vi "Compute if Should Span.vi"(10 "Log Start Time":timestamp, 11 "File Log Specification":T1={"Directory"=path "", "Groups"=[], "Buffer Size"=0, "Properties"=[], "Pretrigger"=FALSE, "Pretrigger Samples"=0, "Name"="", "Timestamp"=FALSE, "Error"=0, "Auto Open"=FALSE, "File Node Ref"=18446744073709551615, "Archive"=FALSE, "Archive Directory"=path "", "Segment Files"=FALSE, "Segment Files By"=enum."Time", "Segment Size"=100000, "Flushed Data Size Total"=0, "Append Waveform Properties"=FALSE, "Logging State"=enum."Not Started", "First Sample Start Time"=timestamp(0 s since 1904-01-01), "System dt"=0.0} {"File Node Ref" format="%.0x"}) -> (3 "Span File":bool)   [LabVIEW 2027, in "Embedded Data Logger Engine.lvlib"]
uses:
  Embedded Data Logger Engine.lvlib
  File Logging Specification.ctl
  Group Logging Specification.ctl
  Group Buffer Data.ctl
  Property Specification.ctl
  <vilib>/NI VeriStand/Custom Device API/Custom Device Item Ref.ctl
  Shared/Segment Files By.ctl
  Logging State.ctl
  <vilib>/NI VeriStand/Custom Device API/Custom Device API.lvlib
  Shared/Embedded Data Logger Shared.lvlib
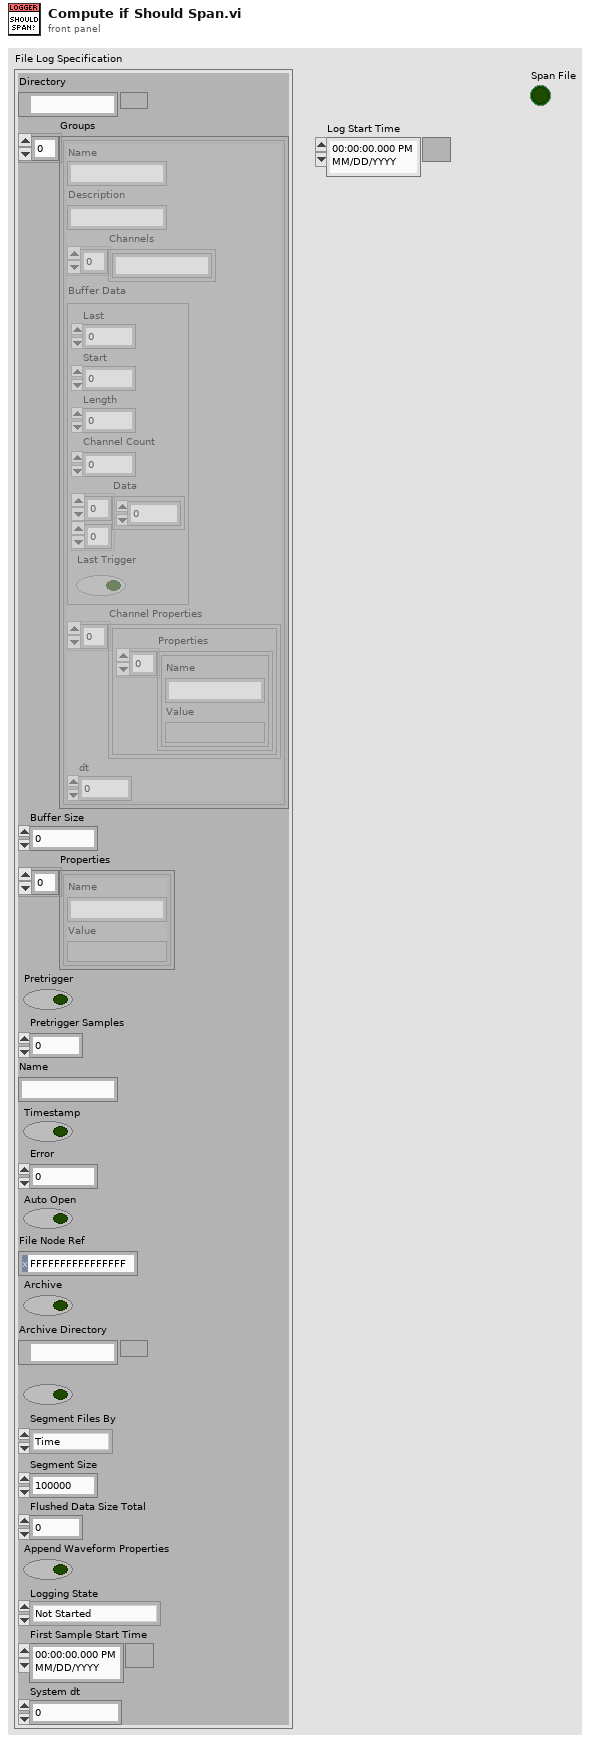
[diagram p1: front panel]
types:
  T1 = typedef "Embedded Data Logger Engine.lvlib/File Logging Specification.ctl" = cluster{"Directory":path, "Groups":T2[], "Buffer Size":i32, "Properties":T4[], "Pretrigger":bool, "Pretrigger Samples":i32, "Name":string, "Timestamp":bool, "Error":i32, "Auto Open":bool, "File Node Ref":T5, "Archive":bool, "Archive Directory":path, "Segment Files":bool, "Segment Files By":T6, "Segment Size":u32, "Flushed Data Size Total":u32, "Append Waveform Properties":bool, "Logging State":T7, "First Sample Start Time":timestamp, "System dt":dbl}
  T2 = typedef "Embedded Data Logger Engine.lvlib/Group Logging Specification.ctl" = cluster{"Name":string, "Description":string, "Channels":string[], "Buffer Data":T3, "Channel Properties":cluster{"Properties":T4[]}[], "dt":dbl}
  T3 = typedef "Embedded Data Logger Engine.lvlib/Group Buffer Data.ctl" = cluster{"Last":i32, "Start":i32, "Length":i32, "Channel Count":i32, "Data":dbl[][], "Last Trigger":bool}
  T4 = typedef "Embedded Data Logger Engine.lvlib/Property Specification.ctl" = cluster{"Name":string, "Value":variant}
  T5 = typedef "Custom Device API.lvlib/Custom Device Item Ref.ctl" = u64
  T6 = typedef "Embedded Data Logger Shared.lvlib/Segment Files By.ctl" = enum16{"Time", "Size"}
  T7 = typedef "Embedded Data Logger Engine.lvlib/Logging State.ctl" = enum16{"Not Started", "Continous Logging", "Paused", "Discontinous Logging"}
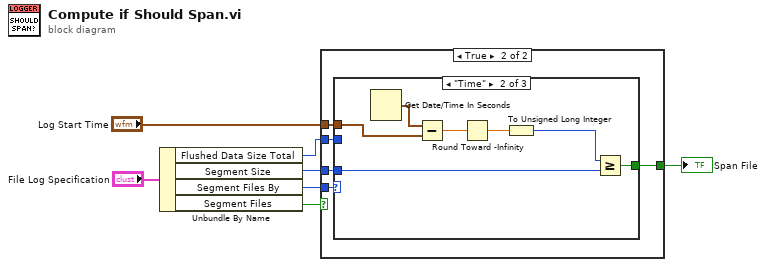
[diagram p0: block diagram]
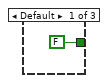
[diagram p3: hidden frame]
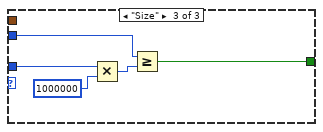
[diagram p4: hidden frame]
diagram:
  n1 = Unbundle By Name("File Log Specification") -> ("Flushed Data Size Total"=w2:u32, "Segment Size"=w3:u32, "Segment Files By"=w6:T6, "Segment Files"=w4:bool)
  n2 = case shown="True" w4 {
    tunnel: w6 -> [_ w12]
    tunnel: w3 -> [_ w11]
    tunnel: [_ w10] -> w5
    tunnel: "Log Start Time" -> [_ w9]
    tunnel: w2 -> [_ w8]
    frame False {
    }
    frame True {
      n3 = case shown="\"Time\"" w12 {
        tunnel: w11 -> [_ w20 w25]
        tunnel: [FALSE w19 w21] -> w10
        tunnel: w9 -> [_ w17 _]
        tunnel: w8 -> [_ _ w22]
        frame Default {
        }
        frame "Time" {
          n4 = Get Date/Time In Seconds() -> (seconds since 1Jan1904=w16:timestamp)
          n5 = Subtract(x=w16, y=w17) -> (x-y=w14:dbl)
          n6 = Round Toward -Infinity(1:w14) -> (0:w15:dbl)
          n7 = To Unsigned Long Integer(number=w15) -> (unsigned 32bit integer=w18:u32)
          n8 = Greater Or Equal?(x=w18, y=w20) -> (x >= y?=w19:bool)
        }
        frame "Size" {
          n9 = Multiply(x=w25, y=u32 1000000 ("x")) -> (x*y=w23:u32)
          n10 = Greater Or Equal?(x=w22, y=w23) -> (x >= y?=w21:bool)
        }
      }
    }
  }
  "Span File" <- w5
